vi "init.vi"(8 "error in (no error)":errorcluster, 11 "Compensator in":refnum<class "SystemController.lvclass">) -> (0 "error out":errorcluster, 3 "Compensator out":refnum<class "SystemController.lvclass">)   [LabVIEW 2013, in "SystemController.lvclass"]
uses:
  SystemController/SystemController.lvclass
  Configuration/SystemController.ctl
  Configuration/ControllerType.ctl
  DualActingPneumaticCylinder_Axial/DualActingPneumaticCylinder_Axial.lvclass
  DualActingPneumaticCylinder_Lateral/DualActingPneumaticCylinder_Lateral.lvclass
  SystemController/SystemController.lvclass/SystemController.ctl
  ConfigurationThisComponent/ConfigurationThisComponent.lvclass
  DualActingPneumaticCylinder/DualActingPneumaticCylinder.lvclass
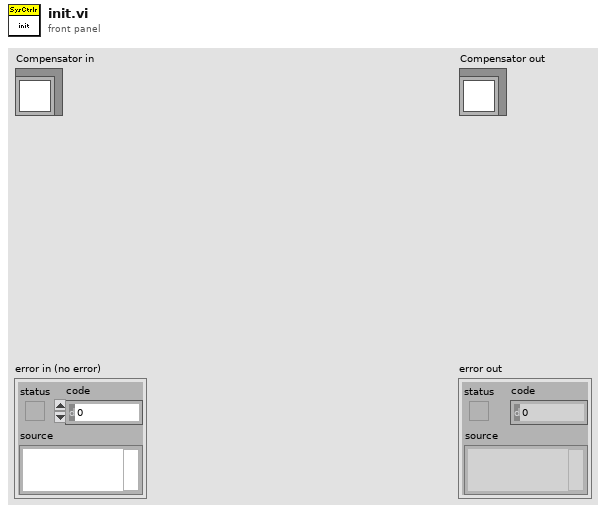
[diagram p1: front panel]
types:
  T1 = typedef "SystemController.ctl" = cluster{"Force Error In Range Limit":dbl[unit], "Controller Type":T2}
  T2 = typedef "ControllerType.ctl" = enum16{"Axial Only", "Axial and Lateral"}
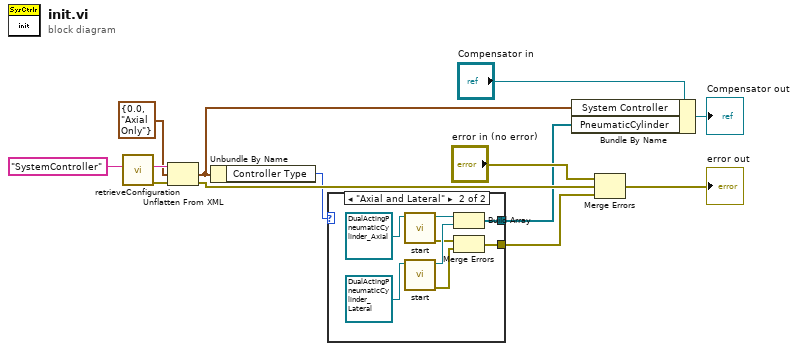
[diagram p0: block diagram]
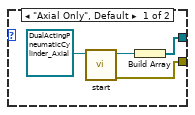
[diagram p2: hidden frame]
diagram:
  n1 = call "retrieveConfiguration.vi"("configName"="SystemController") -> ("error out"=w11:errorcluster, "xmlConfig"=w10:string)  [unwired: 8 in, 1 out]
  n2 = Unflatten From XML(xml string=w10, type=T1 {"Force Error In Range Limit"=0.0, "Controller Type"=enum."Axial Only"} ("Compensator"), error in (no error)=w11) -> (value=w4:T1, error out=w13:errorcluster)
  n3 = Unbundle By Name(w4) -> ("Controller Type"=w3:T2)
  n4 = case shown="\"Axial and Lateral\"" w3 {
    tunnel: [w17 w18] -> w2
    tunnel: [w14 w19] -> w1
    frame "Axial Only", Default {
      n5 = call "start.vi"("DualActingPneumaticCylinder in"=refnum<class "DualActingPneumaticCylinder_Axial.lvclass"> refnum ("DualActingPneumaticCylinder_Axial.lvclass")) -> ("error out"=w14:errorcluster, "DualActingPneumaticCylinder out"=w15:refnum<class "DualActingPneumaticCylinder_Axial.lvclass">)  [unwired: 9 in]
      n6 = Build Array(w15) -> (w17:refnum<class "DualActingPneumaticCylinder_Axial.lvclass">[])
    }
    frame "Axial and Lateral" {
      n7 = call "start.vi"("DualActingPneumaticCylinder in"=refnum<class "DualActingPneumaticCylinder_Axial.lvclass"> refnum ("DualActingPneumaticCylinder_Axial.lvclass")) -> ("error out"=w21:errorcluster, "DualActingPneumaticCylinder out"=w23:refnum<class "DualActingPneumaticCylinder_Axial.lvclass">)  [unwired: 9 in]
      n8 = call "start.vi"("DualActingPneumaticCylinder in"=refnum<class "DualActingPneumaticCylinder_Lateral.lvclass"> refnum ("DualActingPneumaticCylinder_Lateral.lvclass")) -> ("error out"=w20:errorcluster, "DualActingPneumaticCylinder out"=w22:refnum<class "DualActingPneumaticCylinder_Lateral.lvclass">)  [unwired: 9 in]
      n9 = Build Array(w23, w22) -> (w18:refnum<class "DualActingPneumaticCylinder.lvclass">[])
      n10 = Merge Errors(w21, w20) -> (w19:errorcluster)
    }
  }
  n11 = Bundle By Name(cluster="Compensator in", "System Controller"=w4, "PneumaticCylinder"=w2) -> (→"Compensator out":refnum<class "SystemController.lvclass">)
  n12 = Merge Errors("error in (no error)", w13, w1) -> (→"error out":errorcluster)
